vi "Read Configuration Data.vi"(8 "error in":errorcluster, 11 "File Path":path) -> (0 "error out":errorcluster, 1 "VI Title":string, 2 "Configuration Settings":T1, 4 "Panel Colour":u32)   [LabVIEW 2021]
uses:
  controls/Configuration Settings.ctl
  <vilib>/Utility/config.llb/Read Key (I32).vi
  <vilib>/Utility/config.llb/Read Key (Double).vi
  <vilib>/Utility/config.llb/Read Key (String).vi
  <vilib>/Utility/config.llb/Read Key (U32).vi
  <vilib>/Utility/config.llb/NI_LVConfig.lvlib
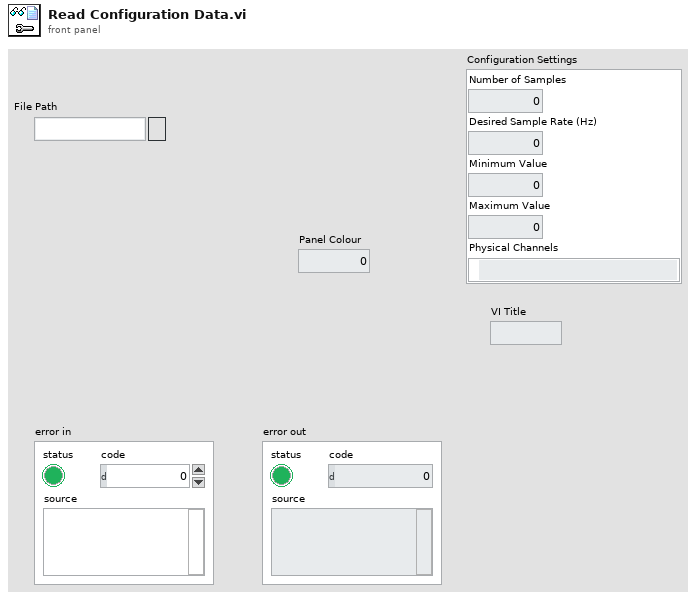
[diagram p1: front panel]
types:
  T1 = typedef "Configuration Settings.ctl" = cluster{"Number of Samples":i32, "Desired Sample Rate (Hz)":dbl, "Minimum Value":dbl, "Maximum Value":dbl, "Physical Channels":tag}
  T2 = typedef "NI_LVConfig.lvlib/Config Data RefNum.ctl" = refnum<k1>
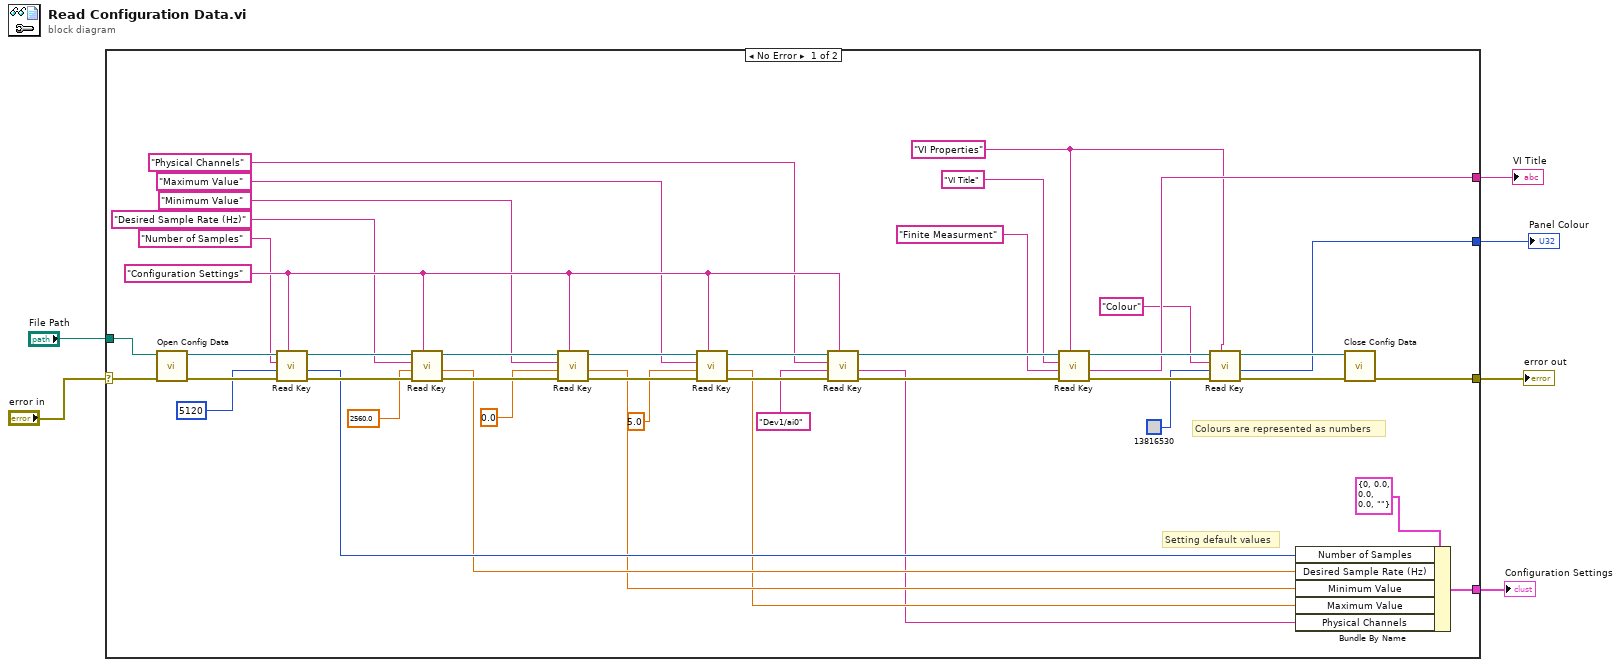
[diagram p0: block diagram]
diagram:
  n1 = case shown="No Error" "error in" {
    selector: "error in" -> [w50 w51]
    tunnel: [w14 w51] -> w5
    tunnel: [w48 _] -> w4
    tunnel: "File Path" -> [w47 _]
    tunnel: [w13 _] -> w2
    tunnel: [w12 _] -> w1
    frame No Error {
      w9 = "VI Properties" ("section")
      w20 = "Configuration Settings"
      # "Colours are represented as numbers"
      # "Setting default values"
      n2 = call <vilib>:"Open Config Data.vi"("error in (no error)"=w50, "configuration file path"=w47) -> ("error out"=w46:errorcluster, "refnum"=w38:T2)  [unwired: 7 in, 1 out]
      n3 = call-poly <vilib>:"Read Key.vi"("section"=w20, "error in (no error)"=w46, "default value"=5120, "key"="Number of Samples", "refnum"=w38) -> ("error out"=w45:errorcluster, "value"=w25:i32, "refnum out"=w37:T2)  [unwired: 3 in, 1 out]
      n4 = call-poly <vilib>:"Read Key.vi"("section"=w20, "error in (no error)"=w45, "default value"=2560.0, "key"="Desired Sample Rate (Hz)", "refnum"=w37) -> ("error out"=w44:errorcluster, "value"=w24:dbl, "refnum out"=w36:T2)  [unwired: 3 in, 1 out]
      n5 = call-poly <vilib>:"Read Key.vi"("section"=w20, "error in (no error)"=w44, "default value"=0.0, "key"="Minimum Value", "refnum"=w36) -> ("error out"=w43:errorcluster, "value"=w23:dbl, "refnum out"=w35:T2)  [unwired: 3 in, 1 out]
      n6 = call-poly <vilib>:"Read Key.vi"("section"=w20, "error in (no error)"=w43, "default value"=5.0, "key"="Maximum Value", "refnum"=w35) -> ("error out"=w42:errorcluster, "value"=w22:dbl, "refnum out"=w34:T2)  [unwired: 3 in, 1 out]
      n7 = call-poly <vilib>:"Read Key.vi"("section"=w20, "error in (no error)"=w42, "default value"="Dev1/ai0", "key"="Physical Channels", "refnum"=w34) -> ("error out"=w41:errorcluster, "value"=w21:string, "refnum out"=w33:T2)  [unwired: 3 in, 1 out]
      n8 = call-poly <vilib>:"Read Key.vi"("section"=w9, "error in (no error)"=w41, "default value"="Finite Measurment", "key"="VI Title", "refnum"=w33) -> ("error out"=w40:errorcluster, "value"=w12:string, "refnum out"=w32:T2)  [unwired: 3 in, 1 out]
      n9 = call-poly <vilib>:"Read Key.vi"("section"=w9, "error in (no error)"=w40, "default value"=u32 13816530, "key"="Colour", "refnum"=w32) -> ("error out"=w39:errorcluster, "value"=w13:u32, "refnum out"=w31:T2)  [unwired: 3 in, 1 out]
      n10 = Bundle By Name(cluster=T1 {"Number of Samples"=0, "Desired Sample Rate (Hz)"=0.0, "Minimum Value"=0.0, "Maximum Value"=0.0, "Physical Channels"=""} ("Configuration Settings"), "Number of Samples"=w25, "Desired Sample Rate (Hz)"=w24, "Minimum Value"=w23, "Maximum Value"=w22, "Physical Channels"=w21) -> (w48:T1)
      n11 = call <vilib>:"Close Config Data.vi"("error in (no error)"=w39, "refnum"=w31) -> ("error out"=w14:errorcluster)  [unwired: 8 in, 1 out]
    }
    frame Error {
    }
  }
  "error out" <- w5
  "VI Title" <- w1
  "Panel Colour" <- w2
  "Configuration Settings" <- w4
